vi "Read (Multiple Responses).vi"(7 "Termination Message ID (-1)":i32=-1, 8 "error in (no error)":errorcluster, 9 "Wait Time Between Responses (3)":u32=3, 11 "VISA resource name":refnum<visa-resource-name>) -> (0 "error out":errorcluster, 1 "Response Bundle Array":T2(array[cluster]), 2 "Response String Array":string[](array[string]), 3 "VISA resource name out":refnum<visa-resource-name>, 4 "First Response Bundle":T1, 5 "Number of Replies":i32)   [LabVIEW 2015, in "Zaber A Series.lvlib"]
doc: "Reads all available responses from the Serial buffer. An array containing the complete strings of the responses is returned on the Response String Array output, and the details of the format of the response are described here: http://www.zaber.com/wiki/Manuals/ASCII_Protocol_Manual#Replies. This VI also parses the strings, bundles the components, and returns them as an array of bundles on the Response Bundle Array pin. Additionally a pin returns the number of responses received. \n\nThis VI requires that the Initialize VI has been called with the same serial port."
uses:
  Zaber A Series.lvlib
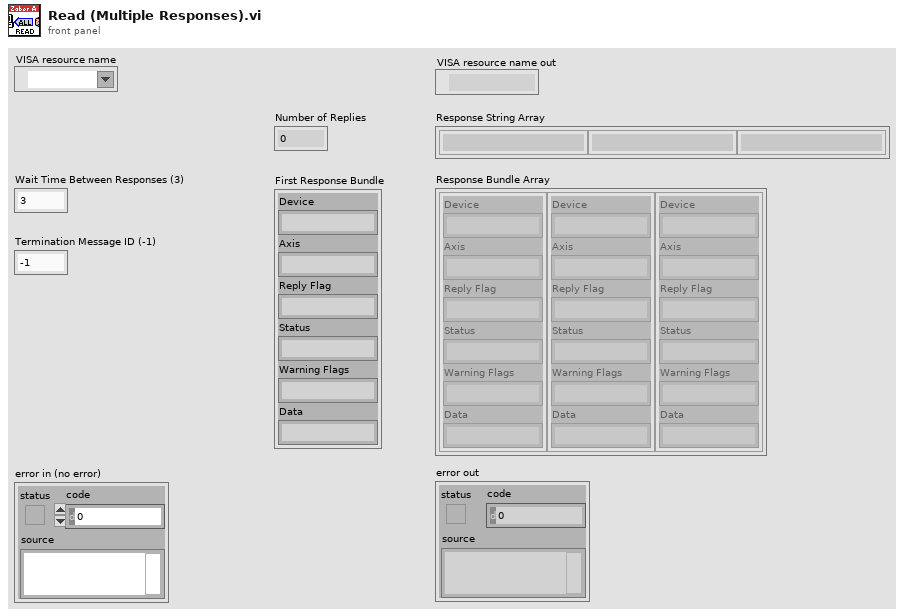
[diagram p1: front panel]
types:
  T1 = cluster{"Device":string, "Axis":string, "Reply Flag":string, "Status":string, "Warning Flags":string, "Data":string}
  T2 = cluster{"Device":string, "Axis":string, "Reply Flag":string, "Status":string, "Warning Flags":string, "Data":string}[]
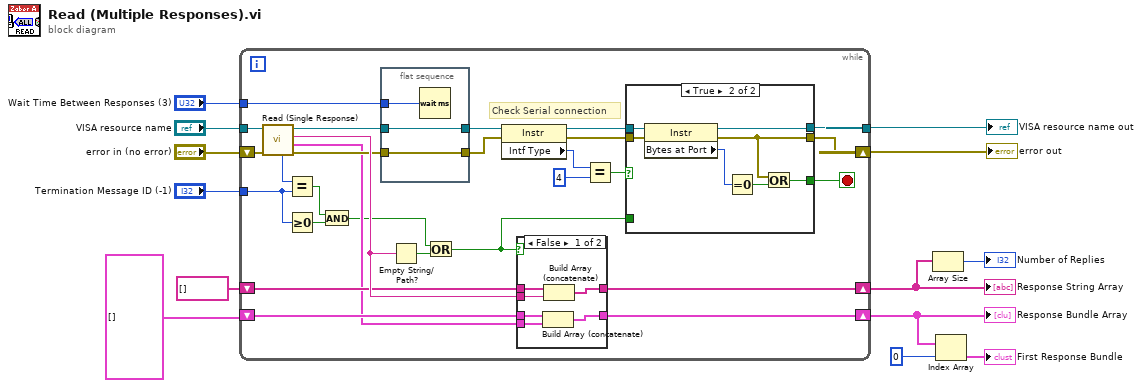
[diagram p0: block diagram]
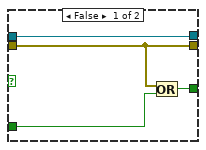
[diagram p2: hidden frame]
diagram:
  n1 = while {
    tunnel: "VISA resource name" -> [w41]
    tunnel: [w24] -> w13
    shift-right: [w38] -> w6
    shift-left: string[] [] -> [w37]
    shift-right: [w36] -> w4
    shift-left: T2 [] -> [w35]
    tunnel: "Wait Time Between Responses (3)" -> [w33]
    shift-right: [w23] -> w12
    shift-left: "error in (no error)" -> [w40]
    tunnel: "Termination Message ID (-1)" -> [w14]
    stop <- w22 stop-if-true
    # "Check Serial connection"
    n2 = call "Read (Single Response).vi"("error in (no error)"=w40, "VISA resource name"=w41) -> ("error out"=w32:errorcluster, "Response Bundle"=w16:T1, "Response"=w39:string, "VISA resource name out"=w34:refnum<visa-resource-name>, "Message ID"=w17:i32)  [unwired: 5 in]
    n3 = Equal?(x=w17, y=w14) -> (x = y?=w18:bool)
    n4 = Greater Or Equal To 0?(x=w14) -> (x >= 0?=w19:bool)
    n5 = And(x=w18, y=w19) -> (x .and. y?=w15:bool)
    n6 = flat-sequence {
      tunnel: w34 -> [w55]
      tunnel: [w55] -> w31
      tunnel: w33 -> [w54]
      tunnel: w32 -> [w53]
      tunnel: [w53] -> w30
      frame #0 {
        n7 = Wait (ms)(milliseconds to wait=w54) -> ()  [unwired: 1 out]
      }
    }
    n8 = Empty String/Path?(string/path=w39) -> (empty?=w21:bool)
    n9 = Or(x=w15, y=w21) -> (x .or. y?=w20:bool)
    n10 = property class="Instr"(reference=w31, error in=w30) -> (reference out=w26:refnum<visa-resource-name>, error out=w25:errorcluster, "Intf Type"=w29:u16)
    n11 = case shown="False" w20 {
      tunnel: w39 -> [w61 _]
      tunnel: [w60 w63] -> w38
      tunnel: w37 -> [w59 w63]
      tunnel: w16 -> [w58 _]
      tunnel: [w57 w62] -> w36
      tunnel: w35 -> [w56 w62]
      frame False {
        n12 = Build Array (concatenate)(w56, w58) -> (w57:T2)
        n13 = Build Array (concatenate)(w59, w61) -> (w60:string[])
      }
      frame True {
      }
    }
    n14 = Equal?(x=w29, y=4) -> (x = y?=w27:bool)
    n15 = case shown="True" w27 {
      tunnel: w26 -> [w45 w52]
      tunnel: w25 -> [w42 w51]
      tunnel: [w45 w49] -> w24
      tunnel: [w44 w47] -> w22
      tunnel: [w42 w46] -> w23
      tunnel: w20 -> [w43 _]
      frame False {
        n16 = Or(x=w42, y=w43) -> (x .or. y?=w44:bool)
      }
      frame True {
        n17 = property class="Instr"(reference=w52, error in=w51) -> (reference out=w49:refnum<visa-resource-name>, error out=w46:errorcluster, "Bytes at Port"=w50:u32)
        n18 = Equal To 0?(x=w50) -> (x = 0?=w48:bool)
        n19 = Or(x=w46, y=w48) -> (x .or. y?=w47:bool)
      }
    }
  }
  "VISA resource name out" <- w13
  "error out" <- w12
  "Response String Array" <- w6
  "Response Bundle Array" <- w4
  n20 = Array Size(array=w6) -> (size(s)=→"Number of Replies":i32)
  n21 = Index Array(array=w4, index=0) -> (element=→"First Response Bundle":T1)
